vi "Tempreture.vi"(10 "Target Temperature":i32=50, 11 "Thermometer  in":i32(slide) scale=0.0..100.0) -> (2 "Checkbox":bool, 3 "Thermometer  out":i32)   [LabVIEW 2021]
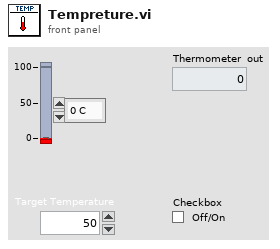
[diagram p1: front panel]
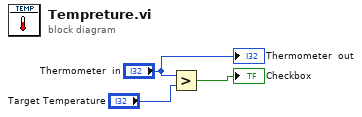
[diagram p0: block diagram]
diagram:
  n1 = Greater?(x="Thermometer  in", y="Target Temperature") -> (0:→"Checkbox":bool)
  "Thermometer  out" <- "Thermometer  in"
